vi "DAC Init Results.vi"(8 "error in":errorcluster, 9 "Log Details?":bool, 10 "tdms file":refnum<k34>, 11 "DAC ADV in":refnum<class "DAC ADV.lvclass">) -> (0 "error out":errorcluster, 2 "tdms file out":refnum<k34>)   [LabVIEW 2019, in "DAC.lvlib" / "DAC ADV.lvclass"]
uses:
  DAC ADV.lvclass
  C:/Users/wg/Documents/LV_Projects/test-stand/App/DAC/DAC.lvclass
  DAC.lvclass/DAC.ctl
  DAC ADV.lvclass/DAC ADV.ctl
  DAC.lvclass
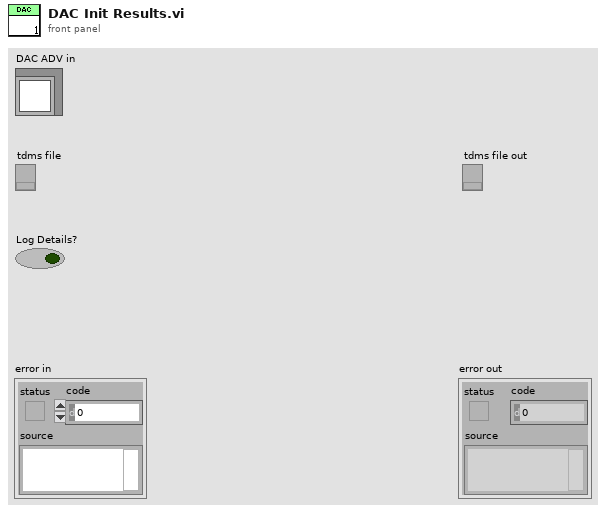
[diagram p1: front panel]
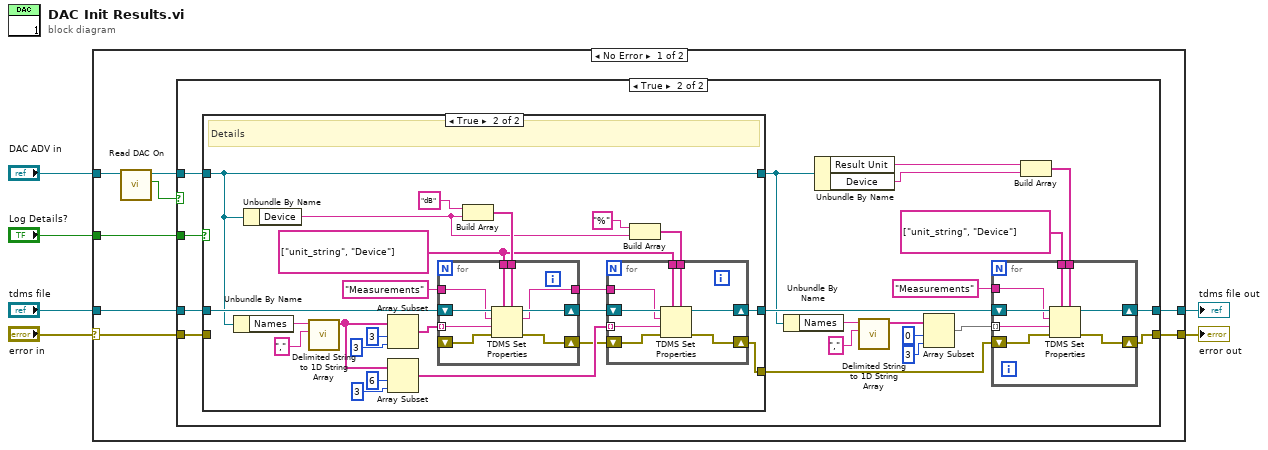
[diagram p0: block diagram]
diagram:
  n1 = case shown="No Error" "error in" {
    selector: "error in" -> [w8 w89]
    tunnel: [w12 w89] -> w3
    tunnel: "DAC ADV in" -> [w11 _]
    tunnel: "tdms file" -> [w14 w88]
    tunnel: [w13 w88] -> w2
    tunnel: "Log Details?" -> [w7 _]
    frame No Error {
      n2 = call "Read DAC On.vi"("DAC in"=w11) -> ("DAC On"=w9:bool, "DAC out"=w10:refnum<class "DAC ADV.lvclass">)  [unwired: 8 in, 1 out]
      n3 = case shown="True" w9 {
        tunnel: w14 -> [w16 w27]
        tunnel: [w16 w35] -> w13
        tunnel: [w15 w34] -> w12
        tunnel: w10 -> [_ w25]
        tunnel: w8 -> [w15 w21]
        tunnel: w7 -> [_ w28]
        frame False {
        }
        frame True {
          n4 = case shown="True" w28 {
            tunnel: w27 -> [w38 w59]
            tunnel: [w38 w46] -> w26
            tunnel: w25 -> [w39 w58]
            tunnel: [w39 w58] -> w24
            tunnel: [w37 w48] -> w22
            tunnel: w21 -> [w37 _]
            frame False {
            }
            frame True {
              w45 = string[] ["unit_string", "Device"] ("property names")
              # "Details"
              n5 = Unbundle By Name(w58) -> ("Names"=w61:string)
              n6 = Unbundle By Name(w58) -> ("Device"=w44:string)
              n7 = call <vilib>:"Delimited String to 1D String Array.vi"("delimiter"=",", "delimited string"=w61) -> ("string array"=w51:string[])  [unwired: 9 in]
              n8 = Array Subset(array=w51, index=3, length=3) -> (w55:string[])
              n9 = Array Subset(array=w51, index=6, length=3) -> (w50:string[])
              n10 = Build Array("dB" ("element"), w44) -> (w60:string[])
              n11 = for {
                tunnel: w45 -> [w78]
                tunnel: w60 -> [w77]
                shift-right: [w76] -> w47
                shift-left: w59 -> [w79]
                tunnel: "Measurements" ("group name in (Untitled)") -> [w74]
                shift-right: [w75] -> w49
                shift-left: _ -> [w73]
                tunnel: w55 -> [w72] mode=indexing
                tunnel: [w71] -> w42
                n12 = TDMS Set Properties(5:w77, 7:w78, 8:w73, 9:w72, 10:w74, 11:w79) -> (0:w75:errorcluster, 2:w71:string, 3:w76:refnum<k34>)  [unwired: 1 out]
              }
              n13 = Build Array("%" ("element"), w44) -> (w43:string[])
              n14 = for {
                tunnel: w45 -> [w69]
                tunnel: w43 -> [w68]
                shift-right: [w67] -> w46
                shift-left: w47 -> [w70]
                tunnel: w42 -> [w65]
                shift-right: [w66] -> w48
                shift-left: w49 -> [w64]
                tunnel: w50 -> [w63] mode=indexing
                n15 = TDMS Set Properties(5:w68, 7:w69, 8:w64, 9:w63, 10:w65, 11:w70) -> (0:w66:errorcluster, 3:w67:refnum<k34>)  [unwired: 2 out]
              }
            }
          }
          n16 = Unbundle By Name(w24) -> ("Names"=w32:string)
          n17 = Unbundle By Name(w24) -> ("Result Unit"=w31:string, "Device"=w29:string)
          n18 = call <vilib>:"Delimited String to 1D String Array.vi"("delimiter"=",", "delimited string"=w32) -> ("string array"=w20:string[])  [unwired: 9 in]
          n19 = Array Subset(array=w20, index=0, length=3) -> (w19:string[])
          n20 = Build Array(w31, w29) -> (w30:string[])
          n21 = for {
            tunnel: w19 -> [w86] mode=indexing
            tunnel: string[] ["unit_string", "Device"] ("property names") -> [w85]
            tunnel: w30 -> [w84]
            shift-right: [w83] -> w35
            shift-left: w26 -> [w87]
            tunnel: "Measurements" ("group name in (Untitled)") -> [w81]
            shift-right: [w82] -> w34
            shift-left: w22 -> [w80]
            n22 = TDMS Set Properties(5:w84, 7:w85, 8:w80, 9:w86, 10:w81, 11:w87) -> (0:w82:errorcluster, 3:w83:refnum<k34>)  [unwired: 2 out]
          }
        }
      }
    }
    frame Error {
    }
  }
  "error out" <- w3
  "tdms file out" <- w2
